vi "Schroeder_Core.vi"(4 "Is output stereo?":bool=TRUE, 6 "Wet(k)":dbl=1.0 min=0.0 max=1.0, 8 "Tail":i32=100 min=0, 9 "Scale N":dbl=1.0 min=0.0, 10 "Scale g":dbl=1.0 min=0.0 format="%#_13g", 11 "Data in (array)":waveform(dbl)[](array[waveform])) -> (3 "Data out (array)":waveform(dbl)[](array[waveform]))   [LabVIEW 2025]
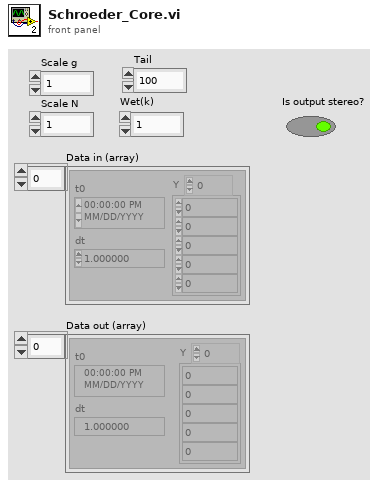
[diagram p1: front panel]
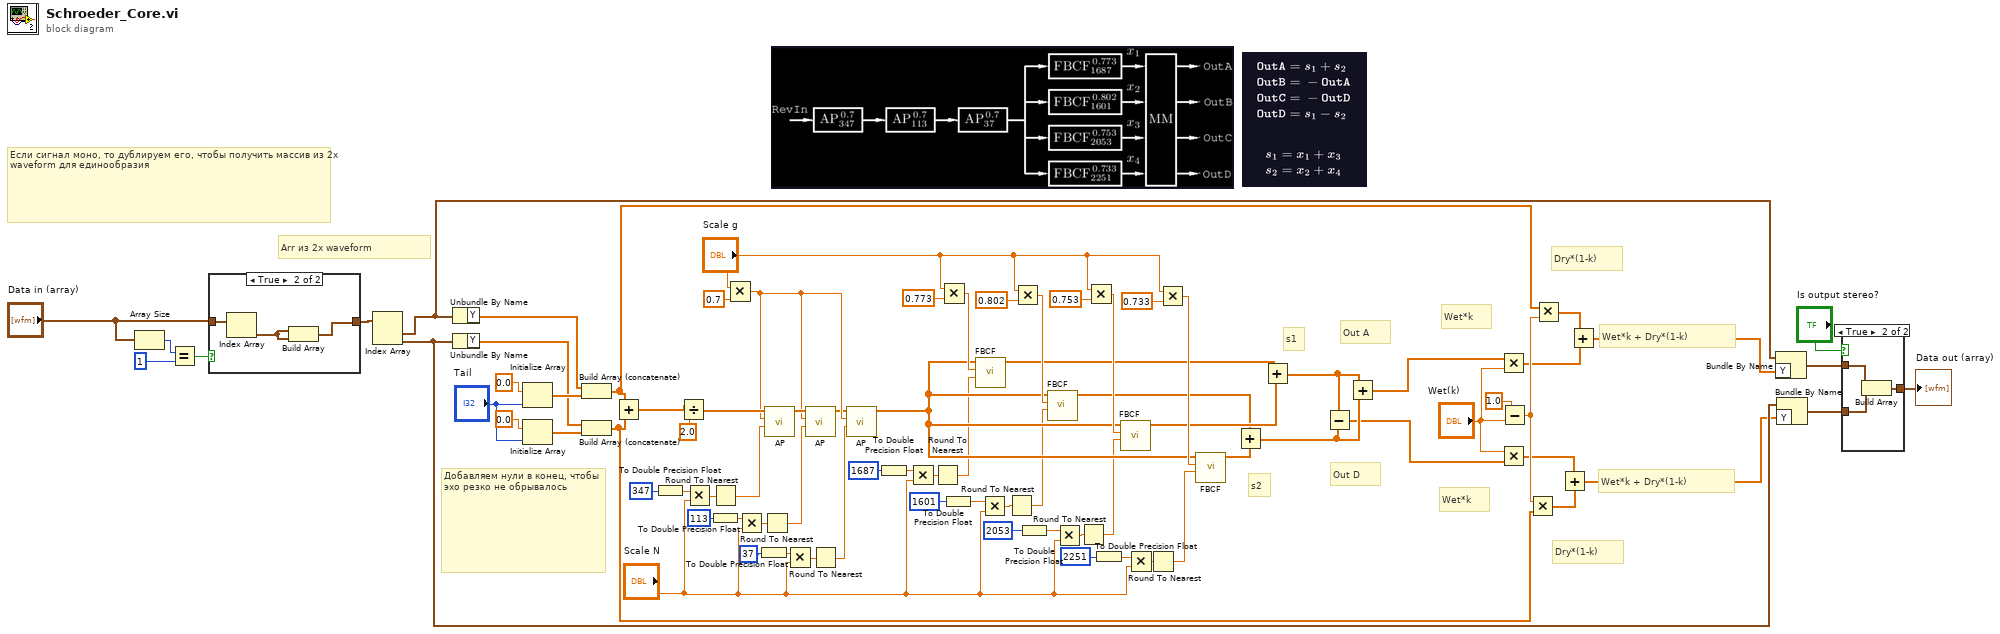
[diagram p0: block diagram]
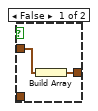
[diagram p2: hidden frame]
diagram:
  # "Wet*k + Dry*(1-k)"
  # "Wet*k + Dry*(1-k)"
  # "Wet*k"
  # "Wet*k"
  # "Dry*(1-k)"
  # "Dry*(1-k)"
  # "Out D"
  # "s2"
  # "s1"
  # "Out A"
  # "Arr из 2х waveform"
  # "Добавляем нули в конец, чтобы эхо резко не обрывалось"
  # "Если сигнал моно, то дублируем его, чтобы получить массив из 2х waveform для единообразия"
  n1 = Array Size(array="Data in (array)") -> (size(s)=w83:i32)
  n2 = Equal?(x=w83, y=1) -> (x = y?=w19:bool)
  n3 = case shown="True" w19 {
    tunnel: "Data in (array)" -> [w84 w87]
    tunnel: [w84 w85] -> w80
    frame False {
    }
    frame True {
      n4 = Index Array(array=w87) -> (element=w86:waveform(dbl))  [unwired: 1 in]
      n5 = Build Array(w86, w86) -> (w85:waveform(dbl)[])
    }
  }
  n6 = Index Array(array=w80) -> (element #1=w34:waveform(dbl), element #2=w33:waveform(dbl))  [unwired: 2 in]
  n7 = Unbundle By Name(w34) -> ("Y"=w74:dbl[])
  n8 = Unbundle By Name(w33) -> ("Y"=w73:dbl[])
  n9 = Initialize Array(0.0 ("element"), "Tail") -> (w75:dbl[])
  n10 = Initialize Array(0.0 ("element"), "Tail") -> (w76:dbl[])
  n11 = Build Array (concatenate)(w74, w75) -> (w26:dbl[])
  n12 = Build Array (concatenate)(w73, w76) -> (w28:dbl[])
  n13 = Add(x=w26, y=w28) -> (x+y=w71:dbl[])
  n14 = To Double Precision Float(number=347 ("Scale N 2")) -> (double precision float=w7:dbl)
  n15 = Divide(x=w71, y=2.0) -> (x/y=w70:dbl[])
  n16 = Multiply(x=w7, y="Scale N") -> (x*y=w52:dbl)
  n17 = Round To Nearest(number=w52) -> (nearest integer value=w14:dbl)
  n18 = To Double Precision Float(number=113 ("Scale N 2")) -> (double precision float=w6:dbl)
  n19 = Multiply(x="Scale g", y=0.7 ("Scale g")) -> (x*y=w54:dbl)
  n20 = Multiply(x=w6, y="Scale N") -> (x*y=w51:dbl)
  n21 = To Double Precision Float(number=37 ("Scale N 2")) -> (double precision float=w5:dbl)
  n22 = Round To Nearest(number=w51) -> (nearest integer value=w13:dbl)
  n23 = call "AP.vi"("N"=w14, "g"=w54, "Data in"=w70) -> ("Data out"=w55:dbl[])  [unwired: 8 in]
  n24 = Multiply(x=w5, y="Scale N") -> (x*y=w50:dbl)
  n25 = call "AP.vi"("N"=w13, "g"=w54, "Data in"=w55) -> ("Data out"=w53:dbl[])  [unwired: 8 in]
  n26 = Round To Nearest(number=w50) -> (nearest integer value=w12:dbl)
  n27 = call "AP.vi"("N"=w12, "g"=w54, "Data in"=w53) -> ("Data out"=w45:dbl[])  [unwired: 8 in]
  n28 = To Double Precision Float(number=1687 ("Scale N 2")) -> (double precision float=w4:dbl)
  n29 = Multiply(x=w4, y="Scale N") -> (x*y=w44:dbl)
  n30 = Round To Nearest(number=w44) -> (nearest integer value=w11:dbl)
  n31 = Multiply(x="Scale g", y=0.773 ("Scale g")) -> (x*y=w49:dbl)
  n32 = To Double Precision Float(number=1601 ("Scale N 2")) -> (double precision float=w3:dbl)
  n33 = call "FBCF.vi"("N"=w11, "g"=w49, "Data in"=w45) -> ("Data out"=w40:dbl[])  [unwired: 8 in]
  n34 = Multiply(x=w3, y="Scale N") -> (x*y=w43:dbl)
  n35 = Round To Nearest(number=w43) -> (nearest integer value=w10:dbl)
  n36 = Multiply(x="Scale g", y=0.802 ("Scale g")) -> (x*y=w46:dbl)
  n37 = To Double Precision Float(number=2053 ("Scale N 2")) -> (double precision float=w2:dbl)
  n38 = call "FBCF.vi"("N"=w10, "g"=w46, "Data in"=w45) -> ("Data out"=w38:dbl[])  [unwired: 8 in]
  n39 = Multiply(x=w2, y="Scale N") -> (x*y=w42:dbl)
  n40 = Round To Nearest(number=w42) -> (nearest integer value=w9:dbl)
  n41 = Multiply(x="Scale g", y=0.753 ("Scale g")) -> (x*y=w48:dbl)
  n42 = To Double Precision Float(number=2251 ("Scale N 2")) -> (double precision float=w1:dbl)
  n43 = call "FBCF.vi"("N"=w9, "g"=w48, "Data in"=w45) -> ("Data out"=w39:dbl[])  [unwired: 8 in]
  n44 = Multiply(x=w1, y="Scale N") -> (x*y=w41:dbl)
  n45 = Round To Nearest(number=w41) -> (nearest integer value=w8:dbl)
  n46 = Multiply(x="Scale g", y=0.733 ("Scale g")) -> (x*y=w47:dbl)
  n47 = call "FBCF.vi"("N"=w8, "g"=w47, "Data in"=w45) -> ("Data out"=w37:dbl[])  [unwired: 8 in]
  n48 = Add(x=w38, y=w37) -> (x+y=w35:dbl[])
  n49 = Add(x=w40, y=w39) -> (x+y=w36:dbl[])
  n50 = Subtract(x=w36, y=w35) -> (x-y=w31:dbl[])
  n51 = Add(x=w36, y=w35) -> (x+y=w32:dbl[])
  n52 = Multiply(x=w32, y="Wet(k)") -> (x*y=w22:dbl[])
  n53 = Multiply(x="Wet(k)", y=w31) -> (x*y=w25:dbl[])
  n54 = Subtract(x=1.0, y="Wet(k)") -> (x-y=w27:dbl)
  n55 = Multiply(x=w27, y=w28) -> (x*y=w24:dbl[])
  n56 = Multiply(x=w26, y=w27) -> (x*y=w23:dbl[])
  n57 = Add(x=w25, y=w24) -> (x+y=w20:dbl[])
  n58 = Add(x=w23, y=w22) -> (x+y=w21:dbl[])
  n59 = Bundle By Name(cluster=w34, "Y"=w21) -> (w17:waveform(dbl))
  n60 = Bundle By Name(cluster=w33, "Y"=w20) -> (w16:waveform(dbl))
  n61 = case shown="True" "Is output stereo?" {
    tunnel: w17 -> [w89 w92]
    tunnel: w16 -> [_ w91]
    tunnel: [w88 w90] -> w15
    frame False {
      n62 = Build Array(w89) -> (w88:waveform(dbl)[])
    }
    frame True {
      n63 = Build Array(w92, w91) -> (w90:waveform(dbl)[])
    }
  }
  "Data out (array)" <- w15
